vi "CRYMultilimit Value Change.vi"(6 "Single Limit":refnum<vi>, 7 "Limits":u16(ring)=2 items=["Upper Only", "Lower Only", "Upper & Lower"], 10 "Multi Limit":refnum<vi>, 11 "Multi value":refnum<vi>) -> (0 "Lo tip":cluster{dbl, dbl}, 1 "Up tip":cluster{dbl, dbl}, 2 "Lower Limit":dbl format="%.2f", 3 "Upper Limit":dbl format="%.2f")   [LabVIEW 2013]
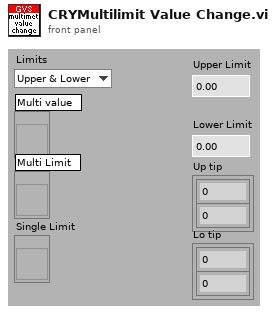
[diagram p1: front panel]
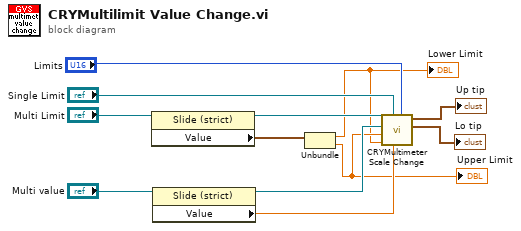
[diagram p0: block diagram]
diagram:
  n1 = property class="Slide (strict)"(reference="Multi Limit") -> (reference out=w10:refnum<vi>, "Value"=w11:cluster{dbl, dbl})  [unwired: 1 in, 1 out]
  n2 = property class="Slide (strict)"(reference="Multi value") -> (reference out=w9:refnum<vi>, "Value"=w8:dbl)  [unwired: 1 in, 1 out]
  n3 = Unbundle(w11) -> (w3:dbl, w4:dbl)
  "Upper Limit" <- w4
  "Lower Limit" <- w3
  n4 = call "CRYMultimeter Scale Change.vi"("Limits"="Limits", "Multi Val"=w8, "Single Limit"="Single Limit", "Low Limit"=w3, "Up Limit"=w4, "Multi value"=w9, "Multi limit"=w10) -> ("Lo tip"=→"Lo tip":cluster{dbl, dbl}, "Up tip"=→"Up tip":cluster{dbl, dbl})  [unwired: 3 out]
